vi "Actor Core.vi"(8 "error in":errorcluster, 11 "UI Controller in":refnum<class "UI Controller.lvclass">) -> (0 "error out":errorcluster, 3 "Actor out":refnum<class "Actor.lvclass">)   [LabVIEW 2020, in "UI Controller.lvlib" / "UI Controller.lvclass"]
uses:
  UI Controller.lvclass
  <vilib>/ActorFramework/Actor/Actor.lvclass
  <vilib>/ActorFrameworkMVC/View Controller/View Controller/View Controller.lvclass
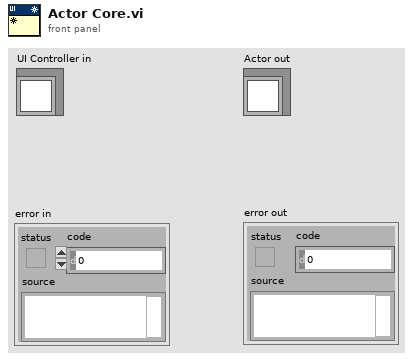
[diagram p1: front panel]
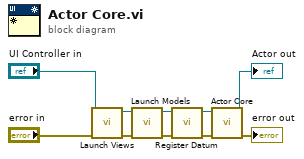
[diagram p0: block diagram]
diagram:
  n1 = call "Launch Views.vi"("error in (no error)"="error in", "UI Controller in"="UI Controller in") -> ("error out"=w7:errorcluster, "UI Controller out"=w8:refnum<class "UI Controller.lvclass">)  [unwired: 8 in]
  n2 = call "Launch Models.vi"("error in (no error)"=w7, "UI Controller in"=w8) -> ("error out"=w5:errorcluster, "UI Controller out"=w6:refnum<class "UI Controller.lvclass">)  [unwired: 8 in]
  n3 = call "Register Datum.vi"("error in (no error)"=w5, "UI Controller in"=w6) -> ("error out"=w2:errorcluster, "UI Controller out"=w1:refnum<class "UI Controller.lvclass">)  [unwired: 8 in]
  n4 = call-parent "Actor Core.vi"("error in"=w2, "Actor in"=w1) -> ("error out"=→"error out":errorcluster, "Actor out"=→"Actor out":refnum<class "Actor.lvclass">)  [unwired: 8 in]
